vi "ReportHead_A131258.vi"(8 "error in (no error)":errorcluster caption="错误输入（无错误）", 11 "产品状态":string) -> (0 "error out":errorcluster caption="错误输出", 3 "report out":refnum<class "NI_report.lvclass"> caption="报表输出")   [LabVIEW 2020]
uses:
  <vilib>/Utility/NIReport.llb/NI_report.lvclass
  <vilib>/addons/_office/_exclsub.llb/font.ctl
  <vilib>/Utility/NIReport.llb/Report Type.ctl
  Database/Global1.vi
  <vilib>/addons/_office/NI_ReportGenerationToolkit.lvlib
  <vilib>/Utility/NIReport.llb/NI_ReportGenerationCore.lvlib
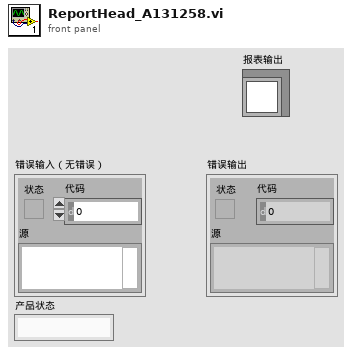
[diagram p1: front panel]
types:
  T1 = typedef "NI_ReportGenerationCore.lvlib/Report Type.ctl" = enum16{"HTML", "Word", "Excel"}
  T2 = cluster{"操作者编号":string, "操作者姓名":string, "操作者权限":string, "联机状态":string, "产品型号":string, "产品状态":string}
  T3 = cluster{"top":dbl, "left":dbl, "right":dbl, "bottom":dbl}
  T4 = cluster{"Charset (-1)":i16, "Weight (-1)":i16, "Name":string, "Size":string}
  T5 = cluster{"Italic":enum16{"Italic Unchanged", "Italic On", "Italic Off"}, "Strike Through":enum16{"Strike Through Unchanged", "Strike Through On", "Strike Through Off"}, "Underline":enum16{"Underline Unchanged", "Underline On", "Underline Off"}, "Bold":enum16{"Bold Unchanged", "Bold On", "Bold Off"}}
  T6 = typedef "NI_ReportGenerationToolkit.lvlib/font.ctl" = cluster{"font name":string, "font size":dbl, "bold":u16, "italic":u16, "underline":u16, "strike through":u16, "font color":u32}
  T7 = enum16{"maximized", "minimized", "normal", "no change"}
  T8 = cluster{"用户编号":string, "用户名":string, "用户密码(密文)":string, "用户权限":string}
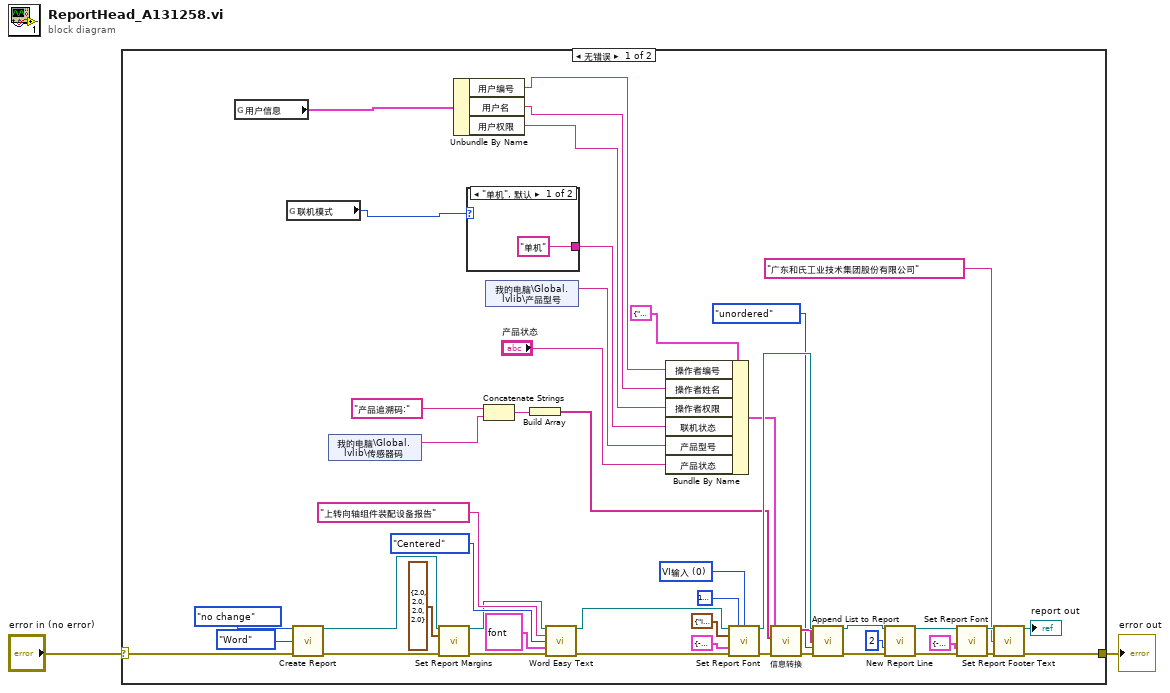
[diagram p0: block diagram]
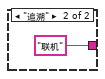
[diagram p2: hidden frame]
diagram:
  n1 = case shown="无错误" "error in (no error)" {
    selector: "error in (no error)" -> [w10 w52]
    tunnel: [w23 w52] -> w1
    frame No Error {
      w44 = u16 0 items=["VI输入", "字体对话框"] ("font settings source")
      n2 = global read "Global1.vi" "用户信息"() -> (w6:T8)
      n3 = global read "Global1.vi" "联机模式"() -> (w7:enum16{"单机", "追溯"})
      n4 = call <vilib>:"Create Report.vi"("window state (normal)"=T7."no change", "report type"=Report_Type."Word", "error in (no error)"=w10) -> ("report out"=w8:refnum<class "NI_report.lvclass">, "error out"=w11:errorcluster)  [unwired: 11 in]
      n5 = shared-variable "我的电脑\\Global.lvlib\\传感器码"() -> (w16:string)  [unwired: 1 in, 1 out]
      n6 = call-dynamic "Set Report Margins.vi"("report in"=w8, "margins (1.00)"=T3 {"top"=2.0, "left"=2.0, "right"=2.0, "bottom"=2.0}, "error in (no error)"=w11) -> ("report out"=w37:refnum<class "NI_report.lvclass">, "error out"=w36:errorcluster)  [unwired: 10 in, 1 out]
      n7 = Unbundle By Name(w6) -> ("用户编号"=w5:string, "用户名"=w4:string, "用户权限"=w3:string)
      n8 = case shown="\"单机\", 默认" w7 {
        tunnel: ["单机" "联机"] -> w20
        frame "单机", Default {
        }
        frame "追溯" {
        }
      }
      n9 = Concatenate Strings("产品追溯码:", w16) -> (w15:string)
      n10 = shared-variable "我的电脑\\Global.lvlib\\产品型号"() -> (w21:string)  [unwired: 1 in, 1 out]
      n11 = Build Array(w15) -> (w14:string[])
      n12 = call <vilib>:"Word Easy Text.vi"("report in"=w37, "text"="上转向轴组件装配设备报告", "alignment (left)"=enum16{"Left", "Centered", "Right", "Justify"}."Centered", "font"=T6 {"font name"="楷体", "font size"=26.0, "bold"=1, "italic"=2, "underline"=2, "strike through"=2, "font color"=16777228}, "error in (no error)"=w36) -> ("report out"=w46:refnum<class "NI_report.lvclass">, "error out"=w45:errorcluster)  [unwired: 8 in, 1 out]
      n13 = Bundle By Name(cluster=T2 {"操作者编号"="001", "操作者姓名"="Administrator", "操作者权限"="系统管理员", "联机状态"="单机", "产品型号"="SL7202", "产品状态"=""} ("测试信息"), "操作者编号"=w5, "操作者姓名"=w4, "操作者权限"=w3, "联机状态"=w20, "产品型号"=w21, "产品状态"="产品状态") -> (w18:T2)
      n14 = call-dynamic "Set Report Font.vi"("report in"=w46, "text color (unchanged)"=u32 16777224, "font settings source (VI Inputs)"=w44, "text options"=T5 {"Italic"=enum."Italic Off", "Strike Through"=enum."Strike Through Unchanged", "Underline"=enum."Underline Off", "Bold"=enum."Bold Off"}, "font settings"=T4 {"Charset (-1)"=-1, "Weight (-1)"=-1, "Name"="微软雅黑 Light", "Size"="12 "}, "error in (no error)"=w45) -> ("report out"=w34:refnum<class "NI_report.lvclass">, "error out"=w26:errorcluster)  [unwired: 7 in, 1 out]
      n15 = call "信息转换.vi"("错误输入（无错误）"=w26, "追溯码"=w14, "测试信息"=w18) -> ("错误输出"=w25:errorcluster, "信息输出"=w27:string[])  [unwired: 7 in]
      n16 = call-dynamic "Append List to Report.vi"("report in"=w34, "list elements"=w27, "list type (ordered)"=enum16{"unordered", "ordered"}."unordered", "error in (no error)"=w25) -> ("report out"=w29:refnum<class "NI_report.lvclass">, "error out"=w28:errorcluster)  [unwired: 8 in, 2 out]
      n17 = call-dynamic "New Report Line.vi"("report in"=w29, "number of lines (1)"=2, "error in (no error)"=w28) -> ("report out"=w32:refnum<class "NI_report.lvclass">, "error out"=w33:errorcluster)  [unwired: 11 in]
      n18 = call-dynamic "Set Report Font.vi"("report in"=w32, "font settings"=T4 {"Charset (-1)"=-1, "Weight (-1)"=-1, "Name"="楷体", "Size"="9 "}, "error in (no error)"=w33) -> ("report out"=w41:refnum<class "NI_report.lvclass">, "error out"=w40:errorcluster)  [unwired: 10 in, 1 out]
      n19 = call-dynamic "Set Report Footer Text.vi"("report in"=w41, "center footer text"="广东和氏工业技术集团股份有限公司", "error in (no error)"=w40) -> ("report out"=→"report out":refnum<class "NI_report.lvclass">, "error out"=w23:errorcluster)  [unwired: 11 in]
    }
    frame Error {
    }
  }
  "error out" <- w1
